vi "Tetromino_RotateRight.vi"(1 "Origin IN":i16, 4 "Tetromino":u8) -> (10 "CheckBorder\nT = RightSide\nF = LeftSide":bool, 15 "Origin OUT":i16, 18 "RotatedTetromino":u8)   [LabVIEW 2018]
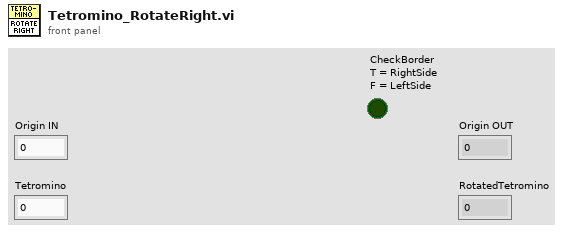
[diagram p1: front panel]
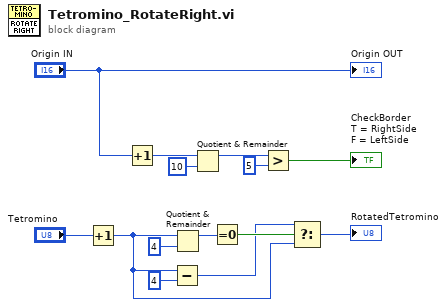
[diagram p0: block diagram]
diagram:
  n1 = Increment(x="Tetromino") -> (x+1=w9:u8)
  n2 = Increment(x="Origin IN") -> (x+1=w6:i16)
  n3 = Subtract(x=w9, y=u8 4) -> (x-y=w10:u8)
  n4 = Quotient & Remainder(x=w9, y=u8 4) -> (x-y*floor(x/y)=w14:u8)  [unwired: 1 out]
  n5 = Quotient & Remainder(x=w6, y=i16 10) -> (x-y*floor(x/y)=w4:i16)  [unwired: 1 out]
  n6 = Equal To 0?(x=w14) -> (x = 0?=w13:bool)
  n7 = Greater?(x=w4, y=i16 5) -> (0:→"CheckBorder\nT = RightSide\nF = LeftSide":bool)
  n8 = Select(t=w10, s=w13, f=w9) -> (s? t:f=→"RotatedTetromino":u8)
  "Origin OUT" <- "Origin IN"
